vi "XML Version.vi"(11 "Data":string) -> (0 "XML Non-Critical Minor":string, 1 "XML Non-Critical Major":string, 2 "XML Critical Minor":string, 3 "XML Critical Major":string)   [LabVIEW 2016, in "GEA2_Toolkit.lvlib"]
uses:
  library/GEA2_Toolkit.lvlib
panel:
  # "03 05 32 00"
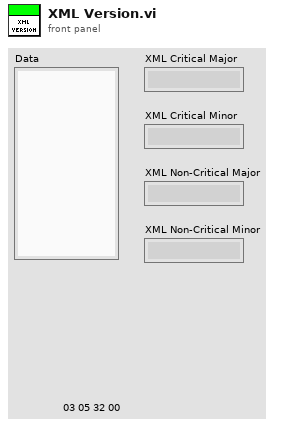
[diagram p1: front panel]
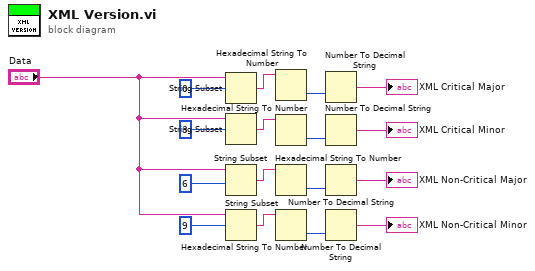
[diagram p0: block diagram]
diagram:
  n1 = String Subset(string="Data", offset (0)=0 ("length (rest)")) -> (substring=w3:string)  [unwired: 1 in]
  n2 = String Subset(string="Data", offset (0)=3 ("length (rest)")) -> (substring=w4:string)  [unwired: 1 in]
  n3 = String Subset(string="Data", offset (0)=6) -> (substring=w7:string)  [unwired: 1 in]
  n4 = String Subset(string="Data", offset (0)=9) -> (substring=w8:string)  [unwired: 1 in]
  n5 = Hexadecimal String To Number(string=w3) -> (number=w5:u32)  [unwired: 2 in, 1 out]
  n6 = Hexadecimal String To Number(string=w4) -> (number=w6:u32)  [unwired: 2 in, 1 out]
  n7 = Hexadecimal String To Number(string=w7) -> (number=w9:u32)  [unwired: 2 in, 1 out]
  n8 = Hexadecimal String To Number(string=w8) -> (number=w12:u32)  [unwired: 2 in, 1 out]
  n9 = Number To Decimal String(number=w5) -> (decimal integer string=→"XML Critical Major":string)  [unwired: 1 in]
  n10 = Number To Decimal String(number=w6) -> (decimal integer string=→"XML Critical Minor":string)  [unwired: 1 in]
  n11 = Number To Decimal String(number=w9) -> (decimal integer string=→"XML Non-Critical Major":string)  [unwired: 1 in]
  n12 = Number To Decimal String(number=w12) -> (decimal integer string=→"XML Non-Critical Minor":string)  [unwired: 1 in]
